vi "getCenter.vi"(8 "ymax":dbl, 9 "ymin":dbl, 10 "xmax":dbl, 11 "xmin":dbl) -> (2 "y":dbl, 3 "x":dbl)   [LabVIEW 2012]
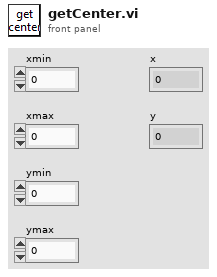
[diagram p1: front panel]
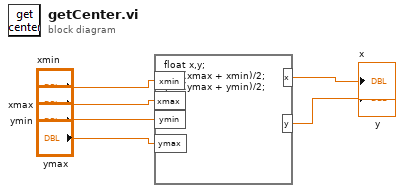
[diagram p0: block diagram]
diagram:
  n1 = formula code="float x,y;\nx = (xmax + xmin)/2;\ny = (ymax + ymin)/2;"("xmin"="xmin", "xmax"="xmax", "ymin"="ymin", "ymax"="ymax") -> ("x"=→"x":dbl, "y"=→"y":dbl)
